vi "Set Active User User Input.vi"(11 "Users":string[](array[string])) -> (0 "Date/Time":string, 3 "Selected User":string)   [LabVIEW 2016]
uses:
  <userlib>/_MGI/Application Control/MGI VI Reference/MGI Current VI's Reference.vi
panel:
  in  "Select the Active User":i32(listbox)
  in  "?":bool
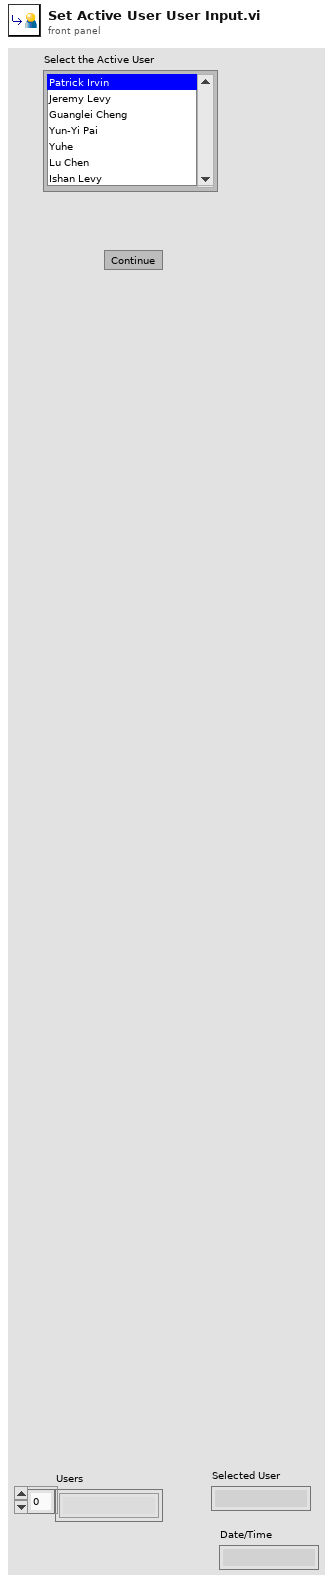
[diagram p1: front panel]
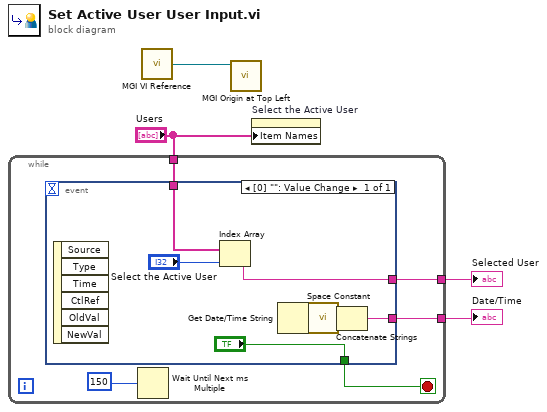
[diagram p0: block diagram]
diagram:
  n1 = while {
    tunnel: [w7] -> w4
    tunnel: "Users" -> [w6]
    tunnel: [w5] -> w1
    stop <- w9 stop-if-true
    n2 = event shown="[0] \"\": Value Change" {
      selector: _ -> [_]
      dyn-events: _ -> [_]
      timeout: _ -> [_]
      tunnel: ["?"] -> w9
      tunnel: [w16] -> w7
      tunnel: w6 -> [w12]
      tunnel: [w10] -> w5
      event Value Change {
        n3 = event-data() -> ()  [unwired: 1 in, 6 out]
        n4 = Index Array(array=w12, index="Select the Active User") -> (element=w10:string)
        n5 = Get Date/Time String() -> (date string=w15:string, time string=w14:string)  [unwired: 3 in]
        n6 = call <vilib>:"Space Constant.vi"() -> ("String"=w13:string)
        n7 = Concatenate Strings(w15, w13, w14) -> (w16:string)
      }
    }
    n8 = Wait Until Next ms Multiple(millisecond multiple=150) -> ()  [unwired: 1 out]
  }
  "Selected User" <- w1
  "Date/Time" <- w4
  n9 = call-poly <userlib>:"MGI VI Reference.vi"() -> ("Current VI's Reference"=w3:refnum<vi>)  [unwired: 1 in]
  n10 = call <userlib>:"MGI Origin at Top Left.vi"("VI Reference In (Caller)"=w3) -> ()  [unwired: 8 in, 2 out]
  n11 = property on="Select the Active User" class="LstBox (strict)"("Item Names"="Users") -> ()  [unwired: 2 in, 2 out]
